vi "Gain into IIR Cluster.vi"(9 "gain":dbl=1.0, 11 "IIR Filter Cluster in":T1 {"Forward Coefficients" format="%.4f"; "Reverse Coefficients" format="%.4f"}) -> (3 "IIR Filter Cluster out":T1 {"Forward Coefficients" format="%.4f"; "Reverse Coefficients" format="%.4f"})   [LabVIEW 2020, in "NI_AALBase.lvlib"]
uses:
  <vilib>/Analysis/NI_AALBase.lvlib
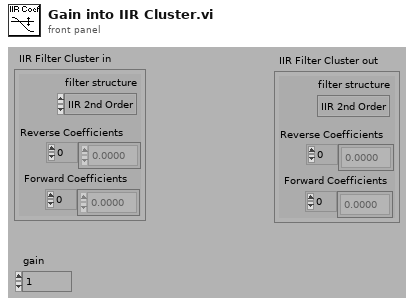
[diagram p1: front panel]
types:
  T1 = cluster{"filter structure":enum32{"IIR 2nd Order", "IIR 4th Order"}, "Reverse Coefficients":dbl[], "Forward Coefficients":dbl[]}
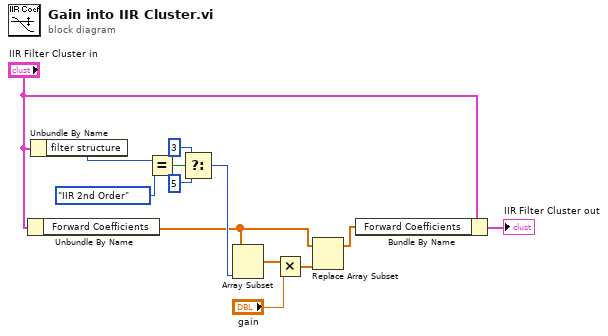
[diagram p0: block diagram]
diagram:
  n1 = Unbundle By Name("IIR Filter Cluster in") -> ("Forward Coefficients"=w2:dbl[])
  n2 = Unbundle By Name("IIR Filter Cluster in") -> ("filter structure"=w12:enum32{"IIR 2nd Order", "IIR 4th Order"})
  n3 = Equal?(x=w12, y=enum32{"IIR 2nd Order", "IIR 4th Order"}."IIR 2nd Order" ("filter structure")) -> (x = y?=w11:bool)
  n4 = Select(t=3, s=w11, f=5 ("t")) -> (s? t:f=w8:i32)
  n5 = Array Subset(array=w2, length=w8) -> (w5:dbl[])  [unwired: 1 in]
  n6 = Multiply(x=w5, y="gain") -> (x*y=w6:dbl[])
  n7 = Replace Array Subset(array=w2, new element=w6) -> (w4:dbl[])  [unwired: 1 in]
  n8 = Bundle By Name(cluster="IIR Filter Cluster in", "Forward Coefficients"=w4) -> (→"IIR Filter Cluster out":T1)
